vi "REQ Initialize Output.vi"(8 "error in (no error)":errorcluster, 9 "DAQ Type":enum16{"Hardware", "Simulation"}(ring), 10 "CAN Output":T1 {"data"."payload" format="%x"; "data"."timestamp" format="%<%.7X\n%x>T"; "data"."type" items=["CAN Data"=0, "CAN Remote"=1, "CAN Bus Error"=2, "CAN 2.0 Data"=8, "CAN FD Data"=16, "CAN FD+BRS Data"=24, "J1939 Data"=192, "Delay"=224, "Log Trigger"=225, "Start Trigger"=226]; "data"."identifier" format="%x"}, 11 "PXI 8513 in":refnum<class "PXI 8513.lvclass">) -> (0 "error out":errorcluster, 3 "PXI 8513 out":refnum<class "PXI 8513.lvclass">)   [LabVIEW 2021, in "CAN.lvlib" / "PXI 8513.lvclass"]
uses:
  PXI 8513.lvclass
  CAN Output.ctl
  <vilib>/xnet/xnet.llb/XNET Frame CAN.ctl
  <vilib>/xnet/xnet.llb/XNET Frame Type CAN.ctl
  PXI 8513.lvclass/PXI 8513.ctl
  <vilib>/xnet/xnet.llb/XNET Create Session (Frame Output Stream).vi
  <resource>/objmgr/xnet.rc
  CAN.lvlib
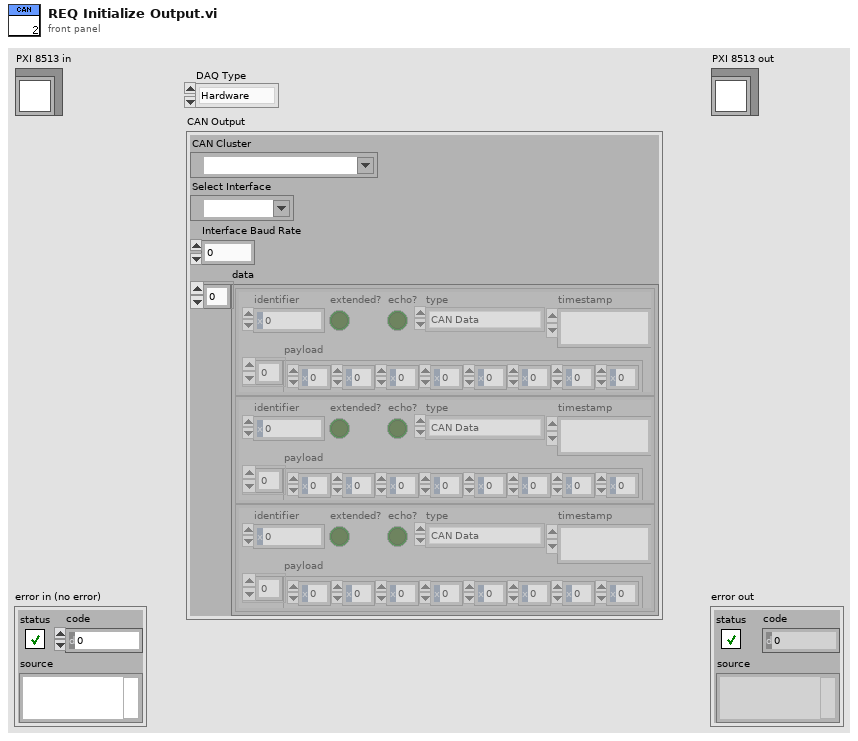
[diagram p1: front panel]
types:
  T1 = typedef "CAN.lvlib/CAN Output.ctl" = cluster{"CAN Cluster":refnum<k21>, "Select Interface":refnum<k21>, "Interface Baud Rate":u32, "data":T2[]}
  T2 = typedef "XNET Frame CAN.ctl" = cluster{"timestamp":timestamp, "payload":u8[], "identifier":u32, "type":T3, "extended?":bool, "echo?":bool}
  T3 = typedef "XNET Frame Type CAN.ctl" = u8
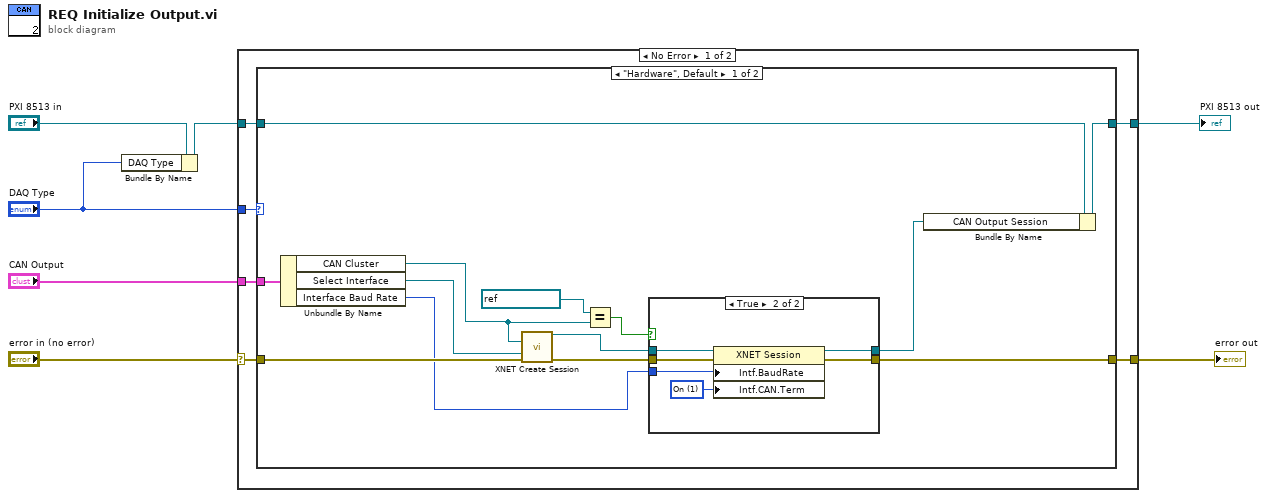
[diagram p0: block diagram]
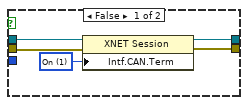
[diagram p2: hidden frame]
diagram:
  n1 = Bundle By Name(cluster="PXI 8513 in", "DAQ Type"="DAQ Type") -> (w6:refnum<class "PXI 8513.lvclass">)
  n2 = case shown="No Error" "error in (no error)" {
    selector: "error in (no error)" -> [w11 w40]
    tunnel: w6 -> [w12 w41]
    tunnel: "DAQ Type" -> [w13 _]
    tunnel: "CAN Output" -> [w10 _]
    tunnel: [w9 w41] -> w2
    tunnel: [w8 w40] -> w1
    frame No Error {
      n3 = case shown="\"Hardware\", Default" w13 {
        tunnel: w12 -> [w17 w39]
        tunnel: w11 -> [w22 w38]
        tunnel: w10 -> [w21 _]
        tunnel: [w16 w39] -> w9
        tunnel: [w14 w38] -> w8
        frame "Hardware", Default {
          n4 = Unbundle By Name(w21) -> ("CAN Cluster"=w20:refnum<k21>, "Select Interface"=w19:refnum<k21>, "Interface Baud Rate"=w18:u32)
          n5 = call-poly <vilib>:"XNET Create Session.vi"("cluster (:memory:)"=w20, "interface"=w19, "error in (no error)"=w22) -> ("session out"=w26:refnum<k21>, "error out"=w25:errorcluster)  [unwired: 11 out]
          n6 = Equal?(x=refnum<k21> ":memory:" ("CAN Cluster"), y=w20) -> (x = y?=w23:bool)
          n7 = case shown="True" w23 {
            tunnel: w26 -> [w30 w37]
            tunnel: [w28 w36] -> w15
            tunnel: w18 -> [_ w35]
            tunnel: [w27 w34] -> w14
            tunnel: w25 -> [w29 w33]
            frame False {
              w31 = u32 1 items=["Off", "On"] ("Interface:CAN:Termination")
              n8 = property class="XNET Session"(reference=w30, error in=w29, "Intf.CAN.Term"=w31) -> (reference out=w28:refnum<k21>, error out=w27:errorcluster)
            }
            frame True {
              w32 = u32 1 items=["Off", "On"] ("Interface:CAN:Termination")
              n9 = property class="XNET Session"(reference=w37, error in=w33, "Intf.BaudRate"=w35, "Intf.CAN.Term"=w32) -> (reference out=w36:refnum<k21>, error out=w34:errorcluster)
            }
          }
          n10 = Bundle By Name(cluster=w17, "CAN Output Session"=w15) -> (w16:refnum<class "PXI 8513.lvclass">)
        }
        frame "Simulation" {
        }
      }
    }
    frame Error {
    }
  }
  "error out" <- w1
  "PXI 8513 out" <- w2
